vi "Build.vi"(8 "error in (no error)":errorcluster, 10 "Root Node":T1) -> (0 "error out":errorcluster)   [LabVIEW 2014, in "CI Project Builder.lvlib"]
uses:
  CI Project Builder.lvlib
  <vilib>/ni/Configuration Framework/Node/NodeRef.ctl
  <vilib>/ni/Configuration Framework/Node/NISE_CEF_Node.lvclass
  Classes/Jenkins Builder/Jenkins Builder.lvclass
  Shared/Classes/Status Updater/Status Updater.lvclass/Status Updater.ctl
  Classes/Jenkins Builder/Jenkins Builder.lvclass/Jenkins Builder.ctl
  <vilib>/ni/Configuration Framework/Node/NISE_CEF_Node.lvclass/NISE_CEF_Node.ctl
  <vilib>/ni/Configuration Framework/Node/ReadChildren.vi
  Shared/Classes/Status Updater/Status Updater.lvclass
  Classes/CI Serializer/CI Serializer.lvclass
panel:
  out "Build Text":string
  out "Progress":u32(slide) scale=0.0..4.0
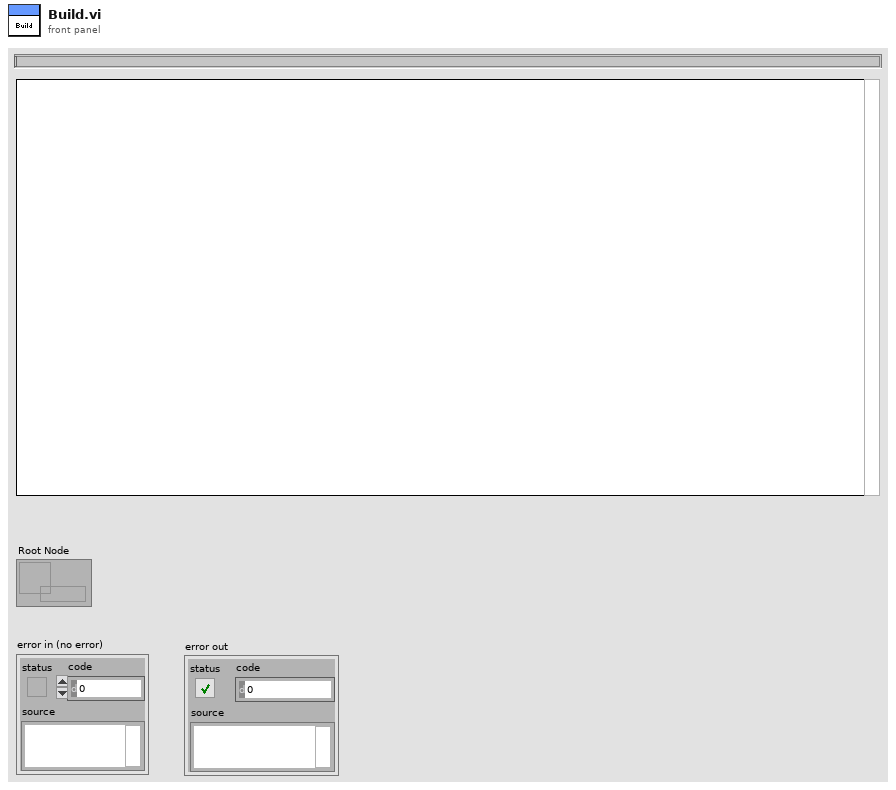
[diagram p1: front panel]
types:
  T1 = typedef "NISE_CEF_Node.lvclass/NodeRef.ctl" = refnum<data-value>
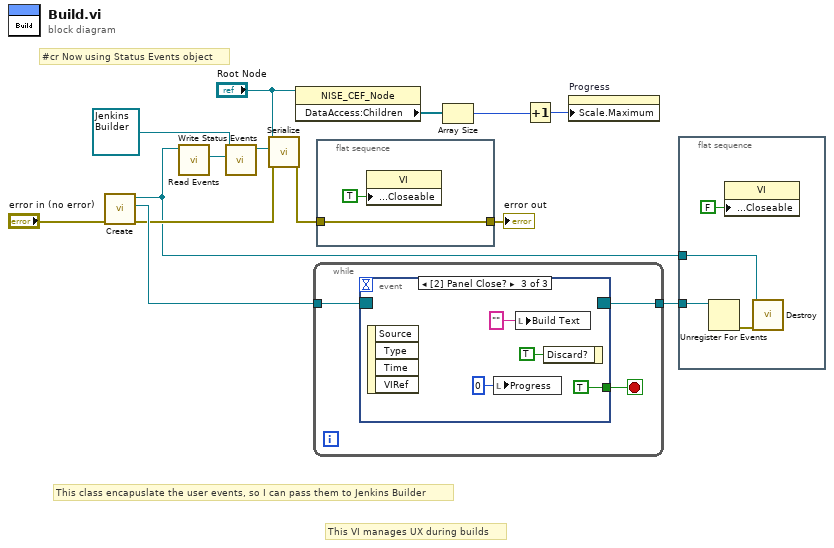
[diagram p0: block diagram]
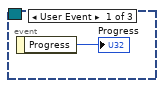
[diagram p2: hidden frame]
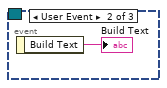
[diagram p3: hidden frame]
diagram:
  # "#cr Now using Status Events object"
  # "This class encapuslate the user events, so I can pass them to Jenkins Builder"
  # "This VI manages UX during builds"
  n1 = call "Create.vi"("error in (no error)"="error in (no error)") -> ("error out"=w9:errorcluster, "Event Registration Refnum"=w10:refnum<event-registration>, "Status Updater out"=w3:refnum<class "Status Updater.lvclass">)  [unwired: 8 in]
  n2 = call "Read Events.vi"("Status Updater in"=w3) -> ("Status Events"=w2:refnum<class "Status Events.lvclass">)  [unwired: 10 in]
  n3 = call "Write Status Events.vi"("Status Events"=w2, "Jenkins Builder in"=refnum<class "Jenkins Builder.lvclass"> refnum ("Jenkins Builder.lvclass")) -> ("Jenkins Builder out"=w11:refnum<class "Jenkins Builder.lvclass">)  [unwired: 9 in]
  n4 = call "Serialize.vi"("error in (no error)"=w9, "CI Serializer in"=w11, "Root Node"="Root Node") -> ("error out"=w8:errorcluster)  [unwired: 7 in, 1 out]
  n5 = property class="NISE_CEF_Node"(reference="Root Node") -> ("DataAccess:Children"=w14:T1[])  [unwired: 1 in, 2 out]
  n6 = while {
    tunnel: w10 -> [w17]
    tunnel: [w15] -> w7
    stop <- w16 stop-if-true
    n7 = event shown="[2] Panel Close?" {
      selector: w17 -> [_ _ _]
      dyn-events: [_ _ _] -> w15
      timeout: _ -> [_ _ _]
      tunnel: [_ _ TRUE ("Front Panel Window:Closeable")] -> w16
      event User Event {
        n8 = event-data() -> ("Progress"=→"Progress":u32)  [unwired: 1 in]
      }
      event User Event {
        n9 = event-data() -> ("Build Text"=→"Build Text":string)  [unwired: 1 in]
      }
      event Panel Close? {
        n10 = event-data() -> ()  [unwired: 1 in, 4 out]
        n11 = local write "Progress"(u32 0 ("Progress")) -> ()
        n12 = local write "Build Text"("") -> ()
        n13 = event-data("Discard?"=TRUE) -> ()  [unwired: 1 in, 1 out]
      }
    }
  }
  n14 = flat-sequence {
    tunnel: w8 -> [w24]
    tunnel: [w24] -> w5
    frame #0 {
      n15 = property class="VI"("Front Panel.Closeable"=TRUE ("Front Panel Window:Closeable")) -> ()  [unwired: 2 in, 2 out]
    }
  }
  n16 = Array Size(array=w14) -> (size(s)=w13:i32)
  n17 = Increment(x=w13) -> (x+1=w4:i32)
  n18 = property on="Progress" class="Slide (strict)"("Scale.Maximum"=w4) -> ()  [unwired: 2 in, 2 out]
  n19 = flat-sequence {
    tunnel: w7 -> [w29]
    tunnel: w3 -> [w27]
    frame #0 {
      n20 = Unregister For Events(event registration refnum=w29) -> (error out=w28:errorcluster)  [unwired: 1 in]
      n21 = property class="VI"("Front Panel.Closeable"=FALSE ("Front Panel Window:Closeable")) -> ()  [unwired: 2 in, 2 out]
      n22 = call "Destroy.vi"("error in (no error)"=w28, "Status Updater in"=w27) -> ()  [unwired: 9 in, 1 out]
    }
  }
  "error out" <- w5
